vi "autonGetIOData.vi"(11 "elapsed auton time":dbl) -> (3 "sensor datas":T1)   [LabVIEW 2012]
panel:
  in  "const":T1
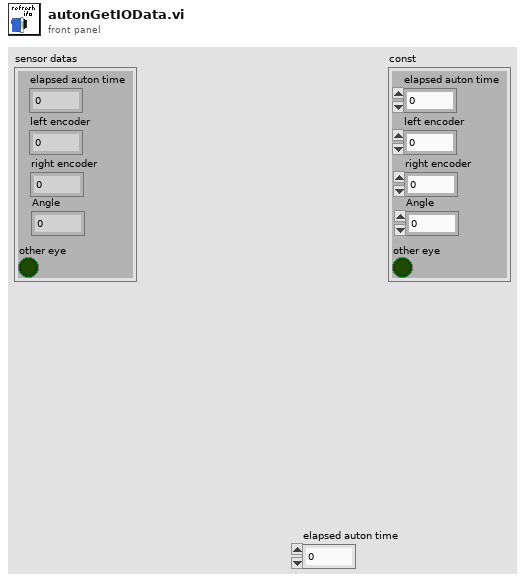
[diagram p1: front panel]
types:
  T1 = cluster{"elapsed auton time":dbl, "left encoder":dbl, "other eye":bool, "right encoder":dbl, "Angle":dbl}
  T2 = typedef "WPI_GyroDevRef.ctl" = cluster{"DevStatus":errorcluster, "Analog Module":T3, "Analog Channel":T4, "Offset":dbl, "Gain (VoltsPerDegree/Second)":dbl}
  T3 = typedef "FPGA_TypedefAnalogModule.ctl" = enum16{"Analog Module 1", "Analog Module 2"}
  T4 = typedef "FPGA_AIChannel.ctl" = enum8{"AI 1", "AI 2", "AI 3", "AI 4", "AI 5", "AI 6", "AI 7", "AI 8", "Invalid"}
  T5 = typedef "WPI_EncoderDevRef.ctl" = cluster{"DevStatus":errorcluster, "EncoderIndex":T6, "CounterIndex":T7, "DistancePerCount":dbl, "Decoding Type":T8}
  T6 = typedef "FPGA_EncoderIdx.ctl" = enum8{"Enc 0", "Enc 1", "Enc 2", "Enc 3", "Invalid"}
  T7 = typedef "FPGA_CounterCtrSystemIndex.ctl" = enum8{"Ctr 0", "Ctr 1", "Ctr 2", "Ctr 3", "Ctr 4", "Ctr 5", "Ctr 6", "Ctr 7", "Invalid"}
  T8 = typedef "WPI_EncoderType.ctl" = enum16{"1x", "2x", "4x"}
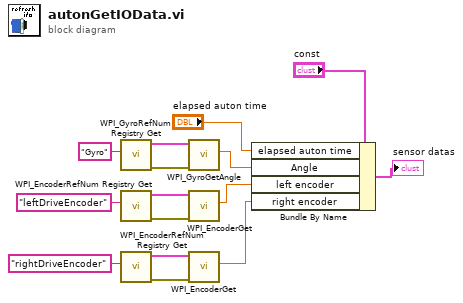
[diagram p0: block diagram]
diagram:
  n1 = call <vilib>:"WPI_GyroRefNum Registry Get.vi"("refnum name"="Gyro") -> ("error out"=w12:errorcluster, "GyroDevRef"=w13:T2)  [unwired: 9 in]
  n2 = call <vilib>:"WPI_EncoderRefNum Registry Get.vi"("refnum name"="leftDriveEncoder") -> ("error out"=w14:errorcluster, "EncoderDevRef"=w15:T5)  [unwired: 9 in]
  n3 = call <vilib>:"WPI_EncoderRefNum Registry Get.vi"("refnum name"="rightDriveEncoder") -> ("error out"=w3:errorcluster, "EncoderDevRef"=w1:T5)  [unwired: 9 in]
  n4 = call <vilib>:"WPI_GyroGetAngle.vi"("error in (no error)"=w12, "GyroDevRef"=w13) -> ("Angle"=w7:dbl)  [unwired: 6 in, 3 out]
  n5 = call <vilib>:"WPI_EncoderGet.vi"("error in (no error)"=w14, "EncoderDevRef"=w15) -> ("Distance"=w5:dbl)  [unwired: 4 in, 5 out]
  n6 = call <vilib>:"WPI_EncoderGet.vi"("error in (no error)"=w3, "EncoderDevRef"=w1) -> ("Distance"=w2:dbl)  [unwired: 4 in, 5 out]
  n7 = Bundle By Name(cluster="const", "elapsed auton time"="elapsed auton time", "Angle"=w7, "left encoder"=w5, "right encoder"=w2) -> (→"sensor datas":T1)
